vi "GSCS_PDA_Client.vi"() -> ()   [LabVIEW 2015]
doc: "Use this template to build a PDA VI for Pocket PC 2002 devices or emulators."
panel:
  in  "connection ID":refnum<k5>
  out "last error":errorcluster
  in  "Exit":bool
  in  "Connect":bool
  # "Goodman Spectrograph \nPDA Interface"
  # "Author:  J Adam Crain\ncrain@physics.unc.edu"
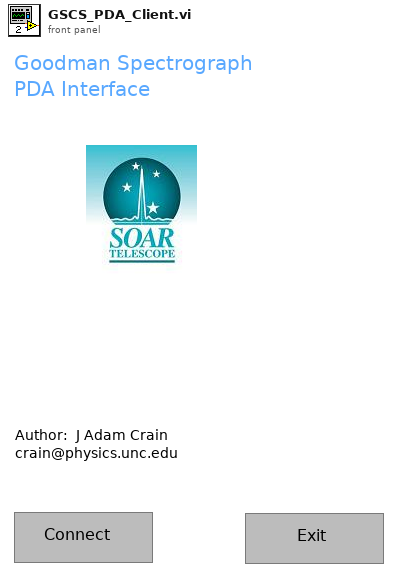
[diagram p1: front panel]
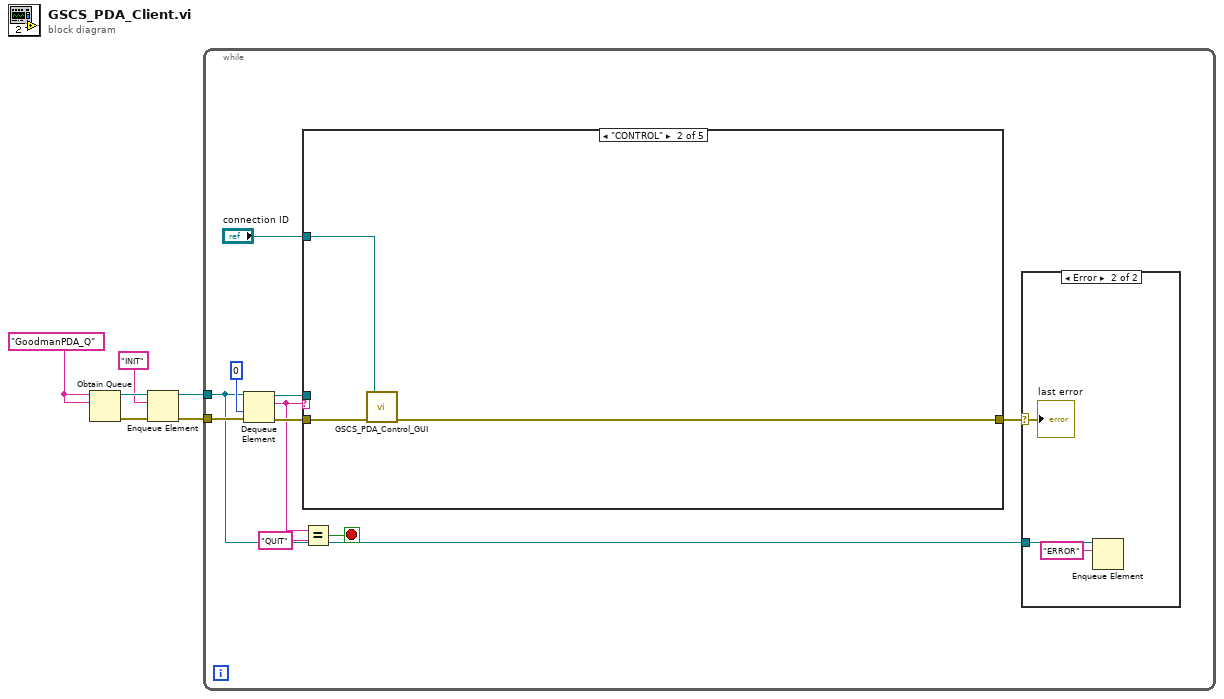
[diagram p0: block diagram]
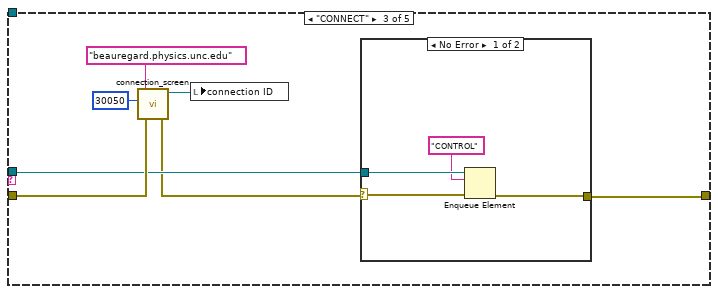
[diagram p4: hidden frame]
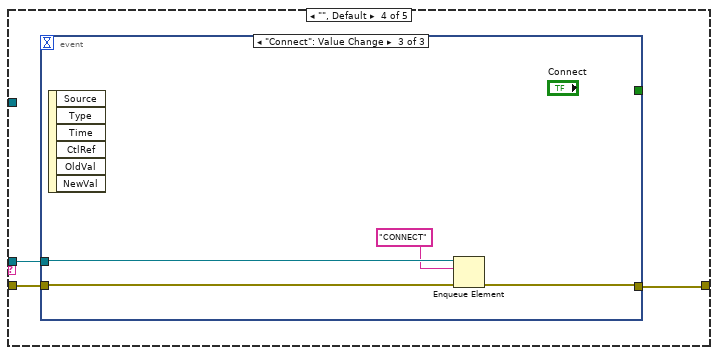
[diagram p6: hidden frame]
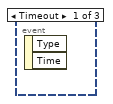
[diagram p7: hidden frame]
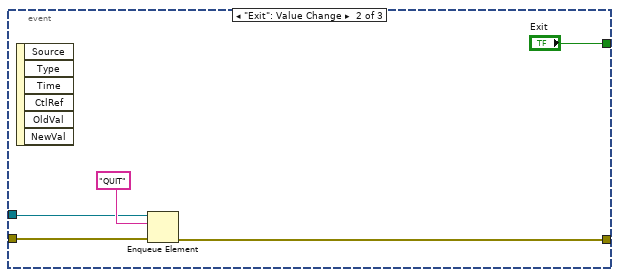
[diagram p8: hidden frame]
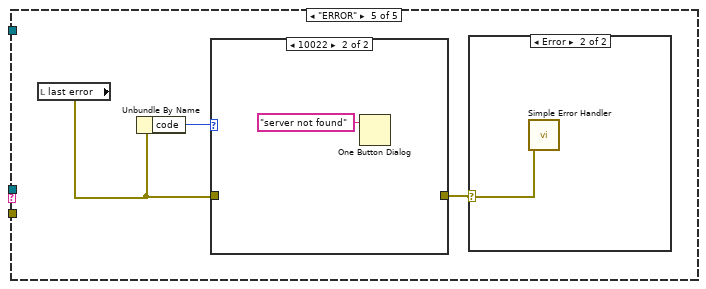
[diagram p9: hidden frame]
diagram:
  w4 = "GoodmanPDA_Q" ("name (unnamed)")
  n1 = Obtain Queue(name (unnamed)=w4, element data type=w4) -> (queue out=w6:refnum<queue>, error out=w5:errorcluster)  [unwired: 3 in, 1 out]
  n2 = Enqueue Element(queue=w6, element="INIT", error in (no error)=w5) -> (queue out=w2:refnum<queue>, error out=w3:errorcluster)  [unwired: 1 in, 1 out]
  n3 = while {
    tunnel: w3 -> [w16]
    tunnel: w2 -> [w8]
    stop <- w10 stop-if-true
    n4 = Dequeue Element(queue=w8, timeout in ms (-1)=0, error in (no error)=w16) -> (queue out=w15:refnum<queue>, element=w12:string, error out=w14:errorcluster)  [unwired: 1 out]
    n5 = case shown="\"CONTROL\"" w12 {
      tunnel: w15 -> [_ _ w28 w38 _]
      tunnel: w14 -> [w20 w23 w30 w37 _]
      tunnel: [w20 w22 w27 w36 _] -> w9
      tunnel: "connection ID" -> [_ w21 _ _ _]
      frame "QUIT" {
      }
      frame "CONTROL" {
        n6 = call "GSCS_PDA_Control_GUI.vi"("error in (no error)"=w23, "TCP Network Connection Refnum"=w21) -> ("error out"=w22:errorcluster)  [unwired: 5 in]
      }
      frame "CONNECT" {
        n7 = call "connection_screen.vi"("error in (no error)"=w30, "remote port"=u16 30050, "address"="beauregard.physics.unc.edu") -> ("error out"=w25:errorcluster, "connection ID"=w26:refnum<k5>)  [unwired: 3 in]
        n8 = local write "connection ID"(w26) -> ()
        n9 = case shown="No Error" w25 {
          selector: w25 -> [w31 w35]
          tunnel: w28 -> [w34 _]
          tunnel: [w32 w35] -> w27
          frame No Error {
            n10 = Enqueue Element(queue=w34, element="CONTROL", error in (no error)=w31) -> (error out=w32:errorcluster)  [unwired: 1 in, 2 out]
          }
          frame Error {
          }
        }
      }
      frame "", Default {
        n11 = event shown="[2] \"Connect\": Value Change" {
          selector: _ -> [_ _ _]
          dyn-events: _ -> [_ _ _]
          timeout: _ -> [_ _ _]
          tunnel: w38 -> [_ w41 w47]
          tunnel: w37 -> [_ w40 w46]
          tunnel: [_ "Exit" _] -> _
          tunnel: [_ w39 w44] -> w36
          event Timeout {
            n12 = event-data() -> ()  [unwired: 1 in, 2 out]
          }
          event "Exit": Value Change {
            n13 = event-data() -> ()  [unwired: 1 in, 6 out]
            n14 = Enqueue Element(queue=w41, element="QUIT", error in (no error)=w40) -> (error out=w39:errorcluster)  [unwired: 1 in, 2 out]
          }
          event "Connect": Value Change {
            n15 = event-data() -> ()  [unwired: 1 in, 6 out]
            n16 = Enqueue Element(queue=w47, element="CONNECT", error in (no error)=w46) -> (error out=w44:errorcluster)  [unwired: 1 in, 2 out]
          }
        }
      }
      frame "ERROR" {
        n17 = local read "last error"() -> (w49:errorcluster)
        n18 = Unbundle By Name(w49) -> ("code"=w50:i32)
        n19 = case shown="10022" w50 {
          tunnel: w49 -> [w52 _]
          tunnel: [w52 _] -> w48
          frame 0, Default {
          }
          frame 10022 {
            n20 = One Button Dialog(message="server not found") -> ()  [unwired: 1 in, 1 out]
          }
        }
        n21 = case shown="Error" w48 {
          selector: w48 -> [_ w51]
          frame No Error {
          }
          frame Error {
            n22 = call <vilib>:"Simple Error Handler.vi"("error in (no error)"=w51) -> ()  [unwired: 4 in, 5 out]
          }
        }
      }
    }
    n23 = Equal?(x=w12, y="QUIT") -> (x = y?=w10:bool)
    n24 = case shown="Error" w9 {
      selector: w9 -> [_ w19]
      tunnel: w8 -> [_ w18]
      frame No Error {
      }
      frame Error {
        n25 = Enqueue Element(queue=w18, element="ERROR") -> ()  [unwired: 2 in, 3 out]
        "last error" <- w19
      }
    }
  }
